vi "JG.vi"(1 "T_W[°C]":dbl, 2 "SHD-PI-02":dbl, 3 "M_manual":dbl) -> (0 "JG [m/s]":dbl)   [LabVIEW 2019]
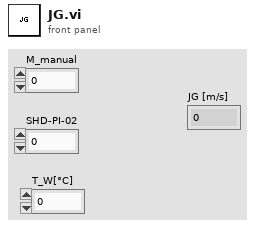
[diagram p1: front panel]
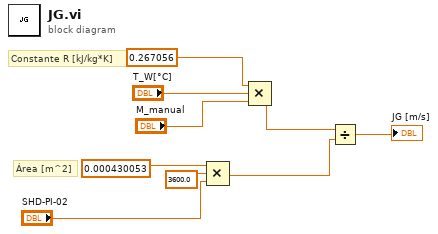
[diagram p0: block diagram]
diagram:
  # "Constante R [kJ/kg*K]"
  # "Área [m^2]"
  n1 = Compound Arithmetic op=MULTIPLY(0.000430053, 3600.0 ("value"), "SHD-PI-02") -> (w4:dbl)
  n2 = Compound Arithmetic op=MULTIPLY(0.267056, "T_W[°C]", "M_manual") -> (w9:dbl)
  n3 = Divide(x=w9, y=w4) -> (x/y=→"JG [m/s]":dbl)
